vi "MarkedRobotStriker.vi"(6 "atacando ao contrário?":bool=TRUE, 8 "Função":T1, 9 "id":u32, 10 "IA State Input":T3={"our_robots"=[], "enemy_robots"=[], "balls"=[], "geometry"={"line_width"=0, "field_length"=0, "field_width"=0, "boundary_width"=0, "referee_width"=0, "goal_width"=0, "goal_depth"=0, "goal_wall_width"=0, "center_circle_radius"=0, "defense_radius"=0, "defense_stretch"=0, "free_kick_from_defense_dist"=0, "penalty_spot_from_field_line_dist"=0, "penalty_line_from_spot_dist"=0}, "IA Judge"={"stage"="", "command"="", "our_goalie_id"=0.0, "enemy_goalie_id"=0.0, "command enum"=enum."Halt", "Time"=enum."Azul"}, "Received Timestamp"=timestamp(0 s since 1904-01-01), "Events"={"Touch"=FALSE, "Ball out"=FALSE, "id touch"=0.0, "Ball out of \nVision"=FALSE, "Ball inside \nGoalie area"=FALSE, "Robot not responding"=FALSE, "Robots responding status"=[1.0, 1.0, 1.0, 1.0, 1.0, 1.0], "Enemy Ball \nPossession"=FALSE, "Pass State"=FALSE, "id end of pass"=0.0, "Kick"=FALSE, "Id ini Possession"=0.0, "Ball Possesion"=FALSE, "Id Possesion"=0.0, "Direct Kick"=FALSE, "2nd Strk Ativo"=FALSE}}, 11 "AI Parameters":T2={"GotoKick"={"Dist do cone a frente"=150.0, "attacker farback"=1500.0, "Perto"=300.0, "min dist to kick"=150.0, "kick eps"=0.0, "Time to transition"=0.05}, "Attacker"={"CC chute"=0.09, "CC passe"=0.045, "Kick Force"=100.0, "ball-robot Kick"=200.0, "ball-robot Pass"=0.3, "drible\nAttk"=FALSE}, "Defender"={"D max"=1700.0, "Vel p/ robô av"=1000.0, "Kick Force"=100.0, "D atk-def"=0.0, "D farback"=0.0, "drible\ndef"=FALSE, "drible\ngoalie"=FALSE}, "Timeout"={"Field/v in x"=6.0, "Dist Robots"=300, "Dist up in y"=300}, "Pose Striker"={"dist"=200.0, "Numeric"=-4.0, "dist 2"=200.0, "drible\nstriker"=FALSE}, "Dist Stop"=300.0, "D ball out"=200, "D central gap "=150.0, "T pass"=0.0, "Force ++"=0.0, "range kick"=0.0, "Chute alto"=TRUE, "Marcador novo"=TRUE, "drible"=FALSE, "D drible"=300.0, "Versão Striker"=enum."3", "Defesa"=enum."ManMark", "Marcador"=enum."Marcar Segundo mais perigoso", "Receptor passe"=enum."2nd Striker", "Área"=enum."Quadrada", "Decisão\nsimples?"=FALSE} {"D drible" format="%#_13g"; "D central gap" format="%#_13g"; "Dist Stop" format="%#_13g"; "Pose Striker"."Numeric" format="%#_13g"; "Defender"."Kick Force" format="%#_13g"; "Defender"."Vel p/ robô av" format="%#_13g"; "Attacker"."ball-robot Kick" format="%#_13g"; "Attacker"."Kick Force" format="%#_13g"; "Attacker"."CC passe" format="%#_13g"; "Attacker"."CC chute" format="%#_13g"; "GotoKick"."kick eps" format="%#_13g"; "GotoKick"."min dist to kick" format="%#_13g"; "GotoKick"."Perto" format="%#_13g"; "GotoKick"."attacker farback" format="%#_13g"; "GotoKick"."Dist do cone a frente" format="%#_13g"}) -> (2 "Dif. tempo\ninimigo bola":dbl, 3 "Robô marcado?":bool=TRUE, 7 "menor dist":dbl)   [LabVIEW 2017]
uses:
  Core/AI Input.ctl
  Core/AI Robot.ctl
  Functions Enum.ctl
  AttackerStates.ctl
  Path Planning/RRT/PathDests.ctl
  Path Planning/RRT/PathDest.ctl
  Core/AI Ball.ctl
  Core/Field Size.ctl
  Core/AI Judge.ctl
  Command Enum.ctl
  Util/Events/Events.ctl
  AI Parameters.ctl
  d3ae8bea-2540-4cab-b848-3da8b8f91e54.vi
  <vilib>/Array/Sort 2D Array - Pop Stack.vi
  <vilib>/Array/Sort 2D Array - Push Stack.vi
panel:
  out "Critério de marcação Normalizado":dbl
  out "Goal Gap Normalizado(%do gol aberta)":dbl
  out "id inimigo \nmaior diferença \nde tempo":dbl
  out "Array":dbl[][](array[numeric])
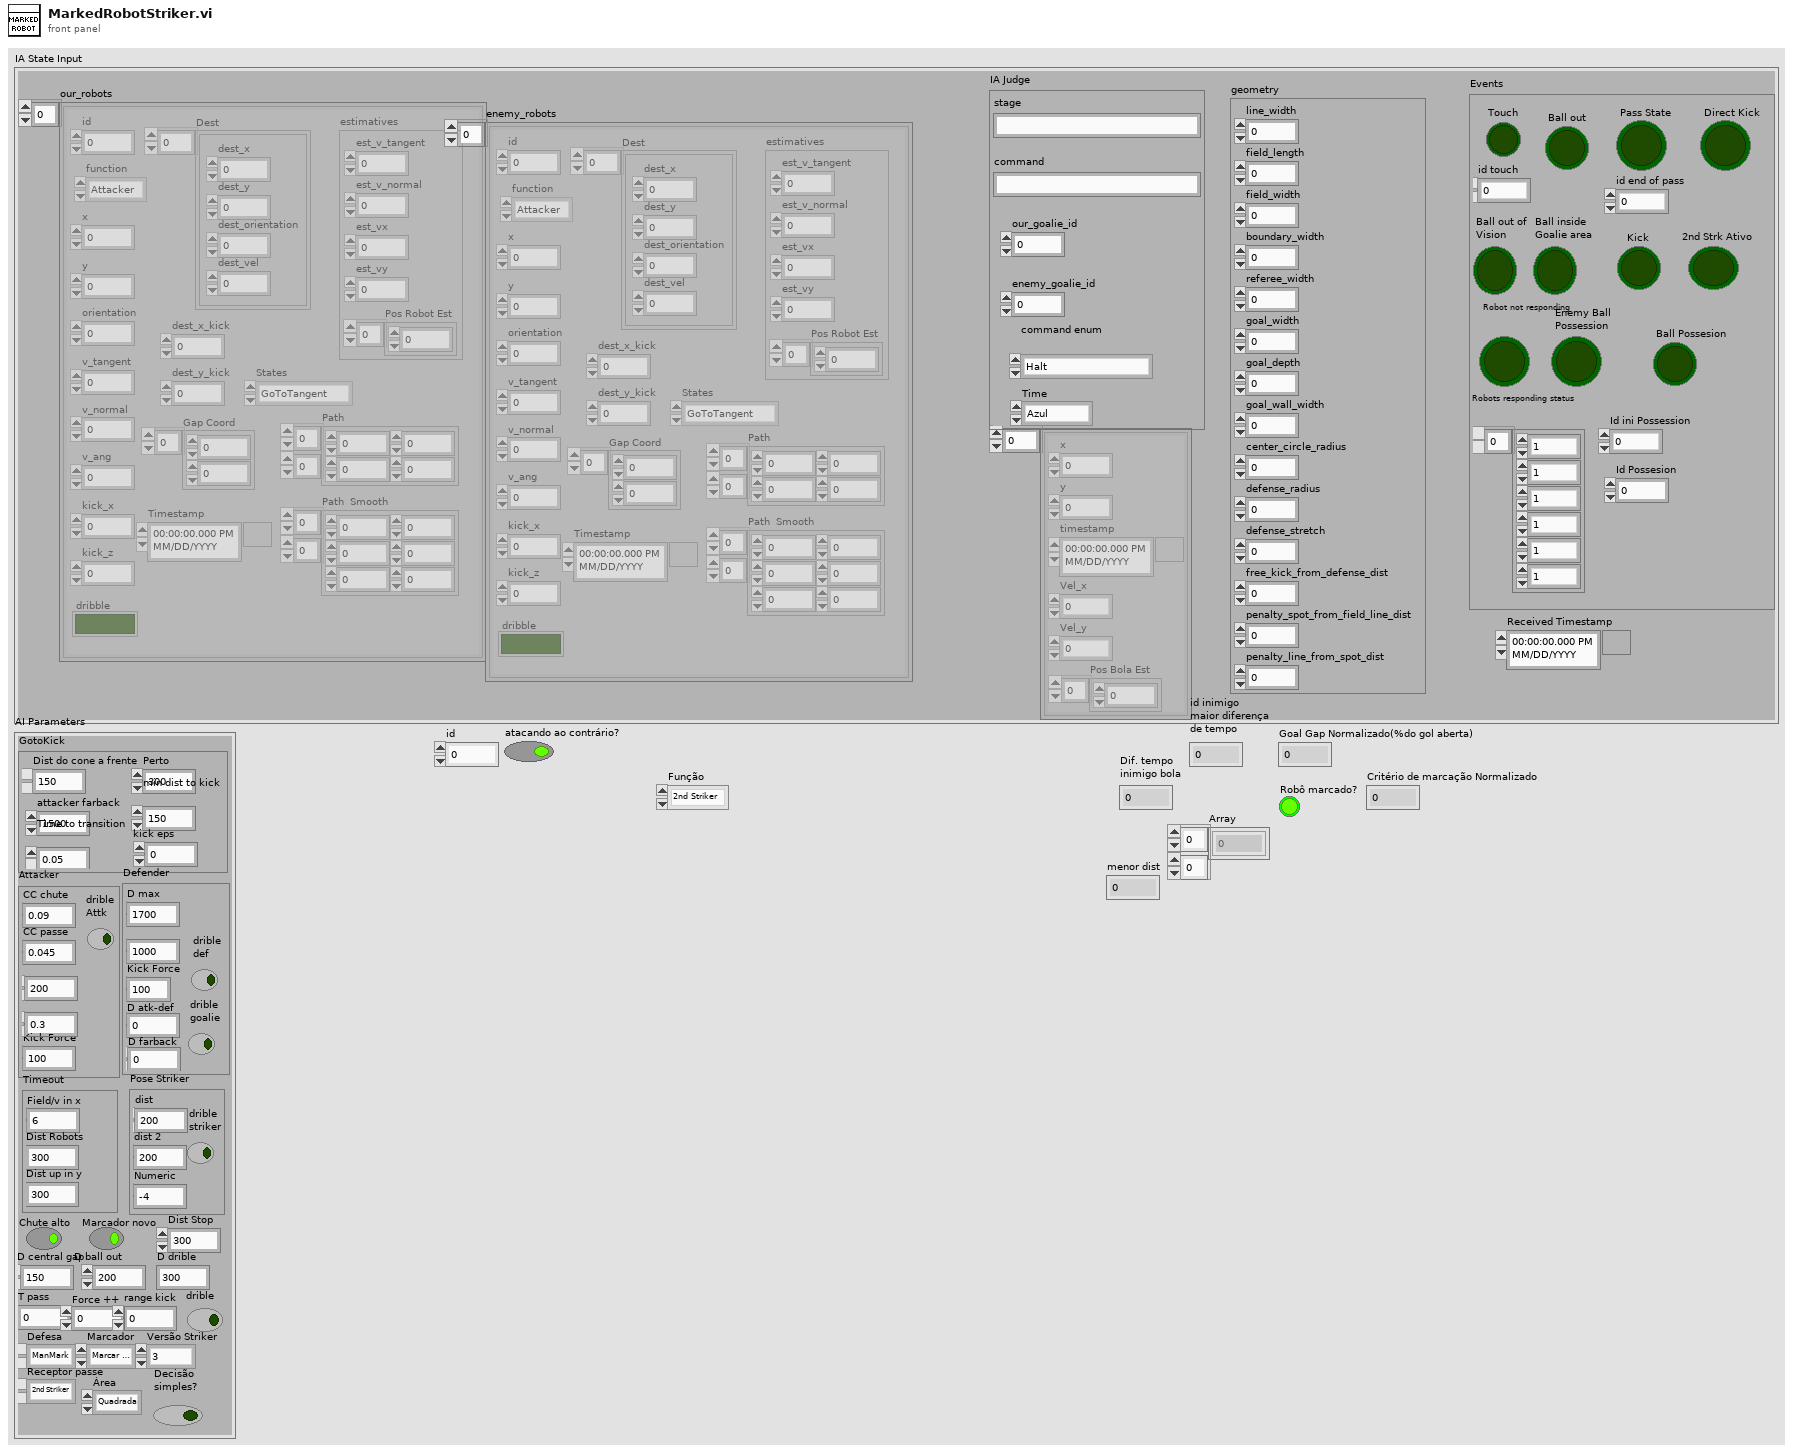
[diagram p1: front panel]
types:
  T1 = typedef "Functions Enum.ctl" = enum16{"2nd Striker", "Attacker", "Goalie", "Defender", "Striker", "Goto 0", "Dummy", "Kicker", "ZigZag 0", "ZigZag 1", "ZigZag 2", "ZigZag 3", "ZigZag 4", "ZigZag 5", "ZigZag 6", "ZigZag 7", "ZigZag 8", ""}
  T2 = typedef "AI Parameters.ctl" = cluster{"GotoKick":cluster{"Dist do cone a frente":dbl, "attacker farback":dbl, "Perto":dbl, "min dist to kick":dbl, "kick eps":dbl, "Time to transition":dbl}, "Attacker":cluster{"CC chute":dbl, "CC passe":dbl, "Kick Force":dbl, "ball-robot Kick":dbl, "ball-robot Pass":dbl, "drible\nAttk":bool}, "Defender":cluster{"D max":dbl, "Vel p/ robô av":dbl, "Kick Force":dbl, "D atk-def":dbl, "D farback":dbl, "drible\ndef":bool, "drible\ngoalie":bool}, "Timeout":cluster{"Field/v in x":dbl, "Dist Robots":u32, "Dist up in y":u32}, "Pose Striker":cluster{"dist":dbl, "Numeric":dbl, "dist 2":dbl, "drible\nstriker":bool}, "Dist Stop":dbl, "D ball out":i32, "D central gap ":dbl, "T pass":dbl, "Force ++":dbl, "range kick":dbl, "Chute alto":bool, "Marcador novo":bool, "drible":bool, "D drible":dbl, "Versão Striker":enum16{"Auto", "3", "2", "1"}, "Defesa":enum16{"ManMark", "Barreira"}, "Marcador":enum16{"Marcar Segundo mais perigoso", "Marcar o mais perigoso"}, "Receptor passe":enum16{"Auto", "2nd Striker", "Striker"}, "Área":enum16{"Quadrada", "Circular"}, "Decisão\nsimples?":bool}
  T3 = typedef "AI Input.ctl" = cluster{"our_robots":T4[], "enemy_robots":T4[], "balls":T8[], "geometry":T9, "IA Judge":T10, "Received Timestamp":timestamp, "Events":T12}
  T4 = typedef "AI Robot.ctl" = cluster{"id":u32, "function":T1, "x":dbl, "y":dbl, "orientation":dbl, "v_tangent":dbl, "v_normal":dbl, "v_ang":dbl, "kick_x":dbl, "kick_z":dbl, "dribble":bool, "Timestamp":timestamp, "estimatives":cluster{"est_v_tangent":dbl, "est_v_normal":dbl, "est_vx":dbl, "est_vy":dbl, "Pos Robot Est":dbl[]}, "dest_x_kick":dbl, "dest_y_kick":dbl, "Gap Coord":dbl[], "States":T5, "Path ":dbl[][], "Path  Smooth":dbl[][], "Dest":T6}
  T5 = typedef "AttackerStates.ctl" = enum16{"Pass", "GoToTangent", "BallGetting", "GoToKick", ""}
  T6 = typedef "PathDests.ctl" = T7[]
  T7 = typedef "PathDest.ctl" = cluster{"dest_x":dbl, "dest_y":dbl, "dest_orientation":dbl, "dest_vel":dbl}
  T8 = typedef "AI Ball.ctl" = cluster{"x":dbl, "y":dbl, "timestamp":timestamp, "Vel_x":dbl, "Vel_y":dbl, "Pos Bola Est":dbl[]}
  T9 = typedef "Field Size.ctl" = cluster{"line_width":u32, "field_length":u32, "field_width":u32, "boundary_width":u32, "referee_width":u32, "goal_width":u32, "goal_depth":u32, "goal_wall_width":u32, "center_circle_radius":u32, "defense_radius":u32, "defense_stretch":u32, "free_kick_from_defense_dist":u32, "penalty_spot_from_field_line_dist":u32, "penalty_line_from_spot_dist":u32}
  T10 = typedef "AI Judge.ctl" = cluster{"stage":string, "command":string, "our_goalie_id":dbl, "enemy_goalie_id":dbl, "command enum":T11, "Time":enum16{"Azul", "Amarelo"}}
  T11 = typedef "Command Enum.ctl" = enum16{"Halt", "Stop", "Force Start", "PKA Normal Start", "Prepare Kickoff Ally", "PKE Normal Start", "Prepare Kickoff Enemy", "Prepare Penalty Ally", "PPA Normal Start", "Prepare Penalty Enemy", "PPE Normal Start", "Direct Free Enemy", "Direct Free Ally", "Indirect Free Enemy", "Indirect Free Ally", "Timeout Enemy", "Timeout Ally", "Goal Enemy", "Goal Ally", "Ball Placement Enemy", "Ball Placement Ally", "Normal Half Time", "Extra Time Break", "Extra Half Time", "None", "Post Game"}
  T12 = typedef "Events.ctl" = cluster{"Touch":bool, "Ball out":bool, "id touch":dbl, "Ball out of \nVision":bool, "Ball inside \nGoalie area":bool, "Robot not responding":bool, "Robots responding status":dbl[], "Enemy Ball \nPossession":bool, "Pass State":bool, "id end of pass":dbl, "Kick":bool, "Id ini Possession":dbl, "Ball Possesion":bool, "Id Possesion":dbl, "Direct Kick":bool, "2nd Strk Ativo":bool}
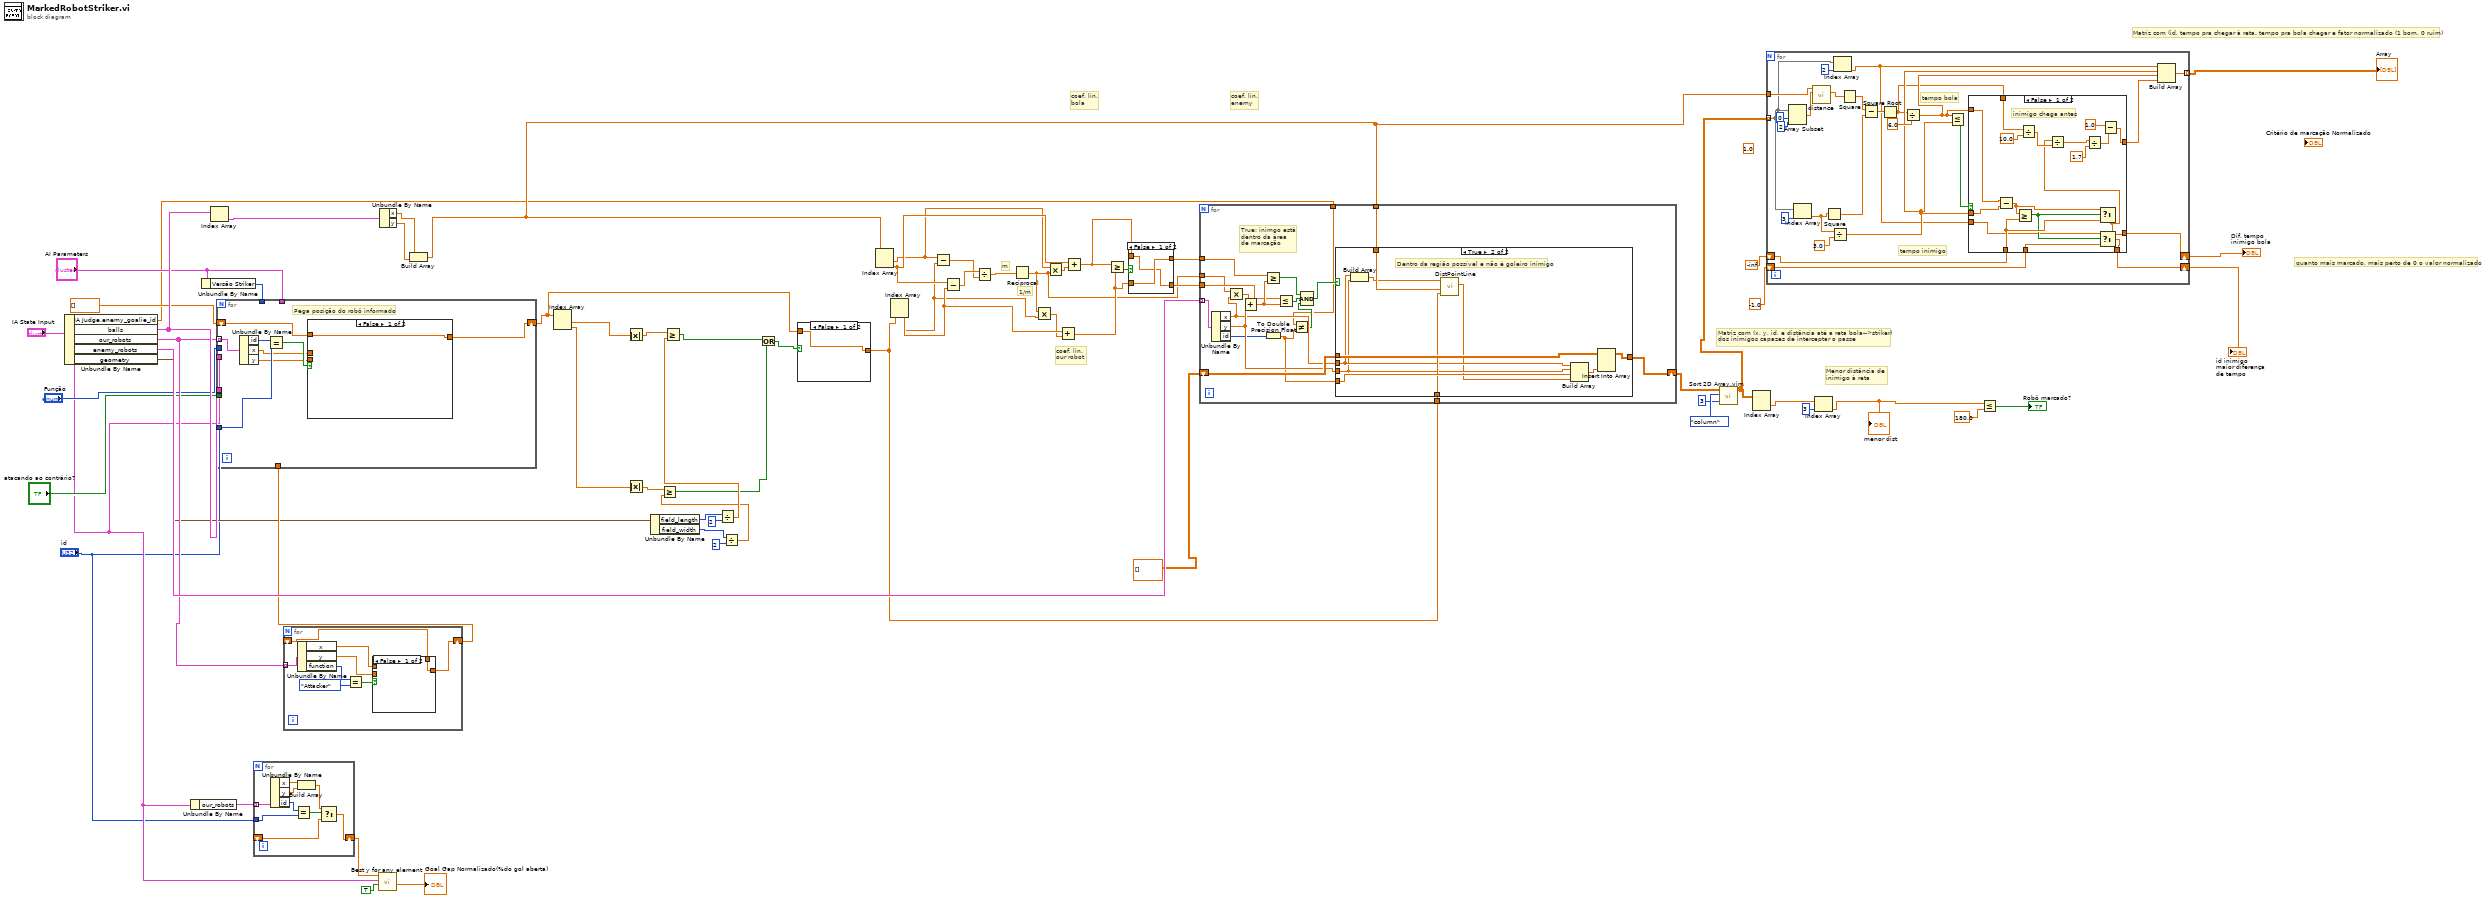
[diagram p0: block diagram]
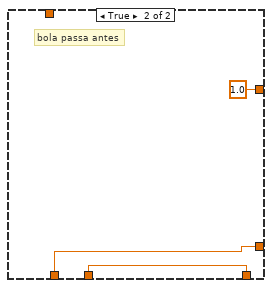
[diagram p2: hidden frame]
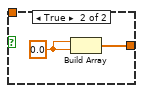
[diagram p3: hidden frame]
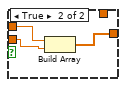
[diagram p4: hidden frame]
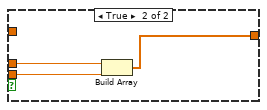
[diagram p7: hidden frame]
diagram:
  (unwired) 1.0
  # "Matriz com (id, tempo pra chegar à reta, tempo pra bola chegar e fator normalizado (1 bom, 0 ruim)"
  # "quanto mais marcado, mais perto de 0 o valor normalizado"
  # "Menor distância de \ninimigo à reta"
  # "Matriz com (x, y, id, e distância até a reta bola-->striker) \ndos inimigos capazes de interceptar o passe"
  # "coef. lin.\nbola"
  # "coef. lin.\nenemy"
  # "coef. lin.\nour robot"
  # "1/m"
  # "m"
  n1 = Unbundle By Name("IA State Input") -> ("IA Judge.enemy_goalie_id"=w1:dbl, "balls"=w45:T8[], "our_robots"=w44:T4[], "enemy_robots"=w58:T4[], "geometry"=w32:T9)
  n2 = Unbundle By Name("IA State Input") -> ("our_robots"=w7:T4[])
  n3 = Unbundle By Name("AI Parameters") -> ("Versão Striker"=w27:enum16{"Auto", "3", "2", "1"})
  n4 = Index Array(array=w45) -> (element=w66:T8)  [unwired: 1 in]
  n5 = for {
    tunnel: w7 -> [w75] mode=indexing
    tunnel: "id" -> [w73]
    shift-right: [w69] -> w5
    shift-left: _ -> [w67]
    n6 = Unbundle By Name(w75) -> ("x"=w72:dbl, "y"=w71:dbl, "id"=w74:u32)
    n7 = Equal?(x=w74, y=w73) -> (x = y?=w68:bool)
    n8 = Build Array(w72, w71) -> (w70:dbl[])
    n9 = Select(t=w70, s=w68, f=w67) -> (s? t:f=w69:dbl[])
  }
  n10 = for {
    tunnel: w44 -> [w83] mode=indexing
    shift-right: [w77] -> w43
    shift-left: _ -> [w76]
    n11 = Unbundle By Name(w83) -> ("x"=w79:dbl, "y"=w78:dbl, "function"=w82:T1)
    n12 = Equal?(x=w82, y=Functions_Enum."Attacker") -> (x = y?=w80:bool)
    n13 = case shown="False" w80 {
      tunnel: w79 -> [_ w87]
      tunnel: w78 -> [_ w86]
      tunnel: [w84 w85] -> w77
      tunnel: w76 -> [w84 _]
      frame False {
      }
      frame True {
        n14 = Build Array(w87, w86) -> (w85:dbl[])
      }
    }
  }
  n15 = for {
    tunnel: w44 -> [w95] mode=indexing
    tunnel: "id" -> [w93]
    shift-right: [w89] -> w9
    shift-left: dbl[] [] -> [w88]
    tunnel: "IA State Input" -> [_]
    tunnel: w45 -> [_]
    tunnel: "AI Parameters" -> [_]
    tunnel: w43 -> [_]
    tunnel: "Função" -> [_]
    tunnel: w27 -> [_]
    tunnel: "atacando ao contrário?" -> [_]
    # "Pega posição do robô informado"
    n16 = Unbundle By Name(w95) -> ("id"=w94:u32, "x"=w91:dbl, "y"=w90:dbl)
    n17 = Equal?(x=w94, y=w93) -> (x = y?=w92:bool)
    n18 = case shown="False" w92 {
      tunnel: w91 -> [_ w99]
      tunnel: w90 -> [_ w98]
      tunnel: [w96 w97] -> w89
      tunnel: w88 -> [w96 _]
      frame False {
      }
      frame True {
        n19 = Build Array(w99, w98) -> (w97:dbl[])
      }
    }
  }
  n20 = call "Best y for any element.vi"("Maior intervalo(T)\nMaior angulo(F)"=TRUE ("Maior intervalo(T)\nMaior angulo(F)"), "IA State"="IA State Input", "Element Position"=w5) -> ("Goal Gap Normalizado(%do gol aberta)"=→"Goal Gap Normalizado(%do gol aberta)":dbl)  [unwired: 4 in, 4 out]
  n21 = Unbundle By Name(w66) -> ("x"=w65:dbl, "y"=w64:dbl)
  n22 = Build Array(w65, w64) -> (w23:dbl[])
  n23 = Index Array(array=w9) -> (element #1=w11:dbl, element #2=w10:dbl)  [unwired: 2 in]
  n24 = Absolute Value(x=w11) -> (abs(x)=w38:dbl)
  n25 = Absolute Value(x=w10) -> (abs(x)=w36:dbl)
  n26 = Unbundle By Name(w32) -> ("field_length"=w42:u32, "field_width"=w39:u32)
  n27 = Divide(x=w42, y=2) -> (x/y=w37:dbl)
  n28 = Greater Or Equal?(x=w38, y=w37) -> (x >= y?=w34:bool)
  n29 = Divide(x=w39, y=u32 2) -> (x/y=w35:dbl)
  n30 = Greater Or Equal?(x=w36, y=w35) -> (x >= y?=w33:bool)
  n31 = Or(x=w34, y=w33) -> (x .or. y?=w31:bool)
  n32 = case shown="False" w31 {
    tunnel: [w100 w101] -> w30
    tunnel: w9 -> [w100 _]
    frame False {
    }
    frame True {
      w102 = 0.0
      n33 = Build Array(w102, w102) -> (w101:dbl[])
    }
  }
  n34 = Index Array(array=w23) -> (element #1=w15:dbl, element #2=w62:dbl)  [unwired: 2 in]
  n35 = Index Array(array=w30) -> (element #1=w16:dbl, element #2=w61:dbl)  [unwired: 2 in]
  n36 = Subtract(x=w15, y=w16) -> (x-y=w59:dbl)
  n37 = Subtract(x=w62, y=w61) -> (x-y=w60:dbl)
  n38 = Divide(x=w60, y=w59) -> (x/y=w63:dbl)
  n39 = Reciprocal(x=w63) -> (1/x=w13:dbl)
  n40 = Multiply(x=w13, y=w16) -> (x*y=w17:dbl)
  n41 = Multiply(x=w15, y=w13) -> (x*y=w14:dbl)
  n42 = Add(x=w61, y=w17) -> (x+y=w55:dbl)
  n43 = Add(x=w62, y=w14) -> (x+y=w56:dbl)
  n44 = Greater Or Equal?(x=w56, y=w55) -> (x >= y?=w57:bool)
  n45 = case shown="False" w57 {
    tunnel: [w104 w106] -> w54
    tunnel: w56 -> [w103 w106]
    tunnel: [w103 w105] -> w53
    tunnel: w55 -> [w104 w105]
    frame False {
    }
    frame True {
    }
  }
  n46 = for {
    tunnel: w58 -> [w125] mode=indexing
    tunnel: w13 -> [w113]
    shift-right: [w123] -> w50
    shift-left: dbl[][] [] -> [w124]
    tunnel: w54 -> [w118]
    tunnel: w53 -> [w117]
    tunnel: w23 -> [w115]
    tunnel: w30 -> [w114]
    tunnel: w1 -> [w108]
    # "True: inimgo está \ndentro da área\nde marcação"
    n47 = Unbundle By Name(w125) -> ("x"=w112:dbl, "y"=w116:dbl, "id"=w110:u32)
    n48 = Multiply(x=w113, y=w112) -> (x*y=w111:dbl)
    n49 = Add(x=w111, y=w116) -> (x+y=w122:dbl)
    n50 = Greater Or Equal?(x=w118, y=w122) -> (x >= y?=w120:bool)
    n51 = To Double Precision Float(number=w110) -> (double precision float=w107:dbl)
    n52 = Less Or Equal?(x=w117, y=w122) -> (x <= y?=w121:bool)
    n53 = Not Equal?(x=w108, y=w107) -> (x != y?=w109:bool)
    n54 = Compound Arithmetic op=AND(w120, w121, w109) -> (w119:bool)
    n55 = case shown="True" w119 {
      tunnel: w124 -> [w126 w136]
      tunnel: [w126 w135] -> w123
      tunnel: w112 -> [_ w130]
      tunnel: w116 -> [_ w129]
      tunnel: w107 -> [_ w134]
      tunnel: w115 -> [_ w132]
      tunnel: w114 -> [_ w131]
      frame False {
        # "Fora da região possível ou é goleiro inimigo"
      }
      frame True {
        # "Dentro da região possível e não é goleiro inimigo"
        n56 = Build Array(w130, w129) -> (w128:dbl[])
        n57 = call "DistPointLine.vi"("P2"=w131, "P1"=w132, "Q"=w128) -> ("distance"=w127:dbl)  [unwired: 8 in]
        n58 = Build Array(w130, w129, w134, w127) -> (w133:dbl[])
        n59 = Insert Into Array(array=w136, new element=w133) -> (w135:dbl[][])  [unwired: 2 in]
      }
    }
  }
  n60 = call "Sort 2D Array.vim"("index"=3, "dimension to index (column)"=enum16{"column", "row"}."column", "2D array"=w50) -> ("sorted 2D array"=w22:dbl[][])  [unwired: 7 in, 1 out]
  n61 = Index Array(array=w22) -> (element=w24:dbl[])  [unwired: 2 in]
  n62 = for {
    tunnel: w23 -> [w144]
    tunnel: w22 -> [w143] mode=indexing
    shift-right: [w139] -> w2
    shift-left: -inf -> [w149]
    tunnel: [w148] -> w20 mode=indexing
    shift-right: [w142] -> w18
    shift-left: -1.0 ("Numeric") -> [w140]
    # "tempo inimigo"
    # "tempo bola"
    n63 = Array Subset(array=w143, index=0, length=2) -> (w158:dbl[])
    n64 = Index Array(array=w143, index=3) -> (element=w152:dbl)
    n65 = call "distance.vi"("P1"=w158, "P2"=w144) -> ("Dist P1P2"=w157:dbl)  [unwired: 9 in]
    n66 = Square(x=w152) -> (x^2=w155:dbl)
    n67 = Divide(x=w152, y=3.0) -> (x/y=w146:dbl)
    n68 = Index Array(array=w143, index=2) -> (element=w141:dbl)
    n69 = Square(x=w157) -> (x^2=w156:dbl)
    n70 = Subtract(x=w156, y=w155) -> (x-y=w154:dbl)
    n71 = Square Root(x=w154) -> (sqrt(x)=w138:dbl)
    n72 = Divide(x=w138, y=6.0) -> (x/y=w147:dbl)
    n73 = Less Or Equal?(x=w147, y=w146) -> (x <= y?=w150:bool)
    n74 = case shown="False" w150 {
      tunnel: w146 -> [w175 _]
      tunnel: w147 -> [w176 _]
      tunnel: [w167 w181] -> w139
      tunnel: w149 -> [w177 w181]
      tunnel: [w173 w180] -> w142
      tunnel: w141 -> [w172 _]
      tunnel: w140 -> [w171 w180]
      tunnel: w138 -> [w170 _]
      tunnel: [w162 1.0] -> w137
      frame False {
        # "inimigo chega antes"
        n75 = Subtract(x=w176, y=w175) -> (x-y=w178:dbl)
        n76 = Greater Or Equal?(x=w178, y=w177) -> (x >= y?=w174:bool)
        n77 = Divide(x=w170, y=10.0) -> (x/y=w168:dbl)
        n78 = Select(t=w178, s=w174, f=w177) -> (s? t:f=w167:dbl)
        n79 = Divide(x=w167, y=w168) -> (x/y=w166:dbl)
        n80 = Divide(x=w166, y=1.7) -> (x/y=w163:dbl)
        n81 = Select(t=w172, s=w174, f=w171) -> (s? t:f=w173:dbl)
        n82 = Subtract(x=1.0, y=w163) -> (x-y=w162:dbl)
      }
      frame True {
        # "bola passa antes"
      }
    }
    n83 = Build Array(w141, w146, w147, w137) -> (w148:dbl[])
  }
  "Dif. tempo\ninimigo bola" <- w2
  "Array" <- w20
  "id inimigo \nmaior diferença \nde tempo" <- w18
  n84 = Index Array(array=w24, index=3) -> (element=w25:dbl)
  "menor dist" <- w25
  n85 = Less Or Equal?(x=w25, y=180.0) -> (x <= y?=→"Robô marcado?":bool)
